vi "Merge Error.vi"(10 "Error":errorcluster, 11 "Set Error in":refnum<class "Dev Panel.lvclass">) -> (3 "Set Error out":refnum<class "Dev Panel.lvclass">)   [LabVIEW 2021, in "Dev Panel.lvclass"]
uses:
  Dev Panel.lvclass
  Dev Panel.lvclass/Dev Panel.ctl
  Actor/Event Actor/Event Actor.lvclass
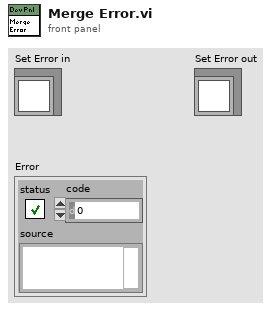
[diagram p1: front panel]
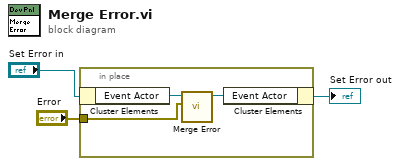
[diagram p0: block diagram]
diagram:
  n1 = in-place {
    in-place-border: "Error" -> [w6]
    n2 = in-place-cluster #1("Set Error in") -> ("Event Actor"=w5:refnum<class "Event Actor.lvclass">)
    n3 = call-dynamic "Merge Error.vi"("Error"=w6, "Set Error in"=w5) -> ("Set Error out"=w4:refnum<class "Event Actor.lvclass">)  [unwired: 9 in]
    n4 = in-place-cluster #1("Event Actor"=w4) -> (→"Set Error out":refnum<class "Dev Panel.lvclass">)
  }
